vi "Time.vi"(8 "error in (no error)":errorcluster, 10 "Control In":T1={"I-O.lvclass"=refnum, "Motion.lvclass"=refnum, "Dispenser.lvclass"=refnum}, 11 "C4 Dispense in":refnum<class "Iterative Dispense.lvclass">) -> (0 "error out":errorcluster, 1 "Timing Data":i32[](array[numeric]), 2 "Control Out":T1, 3 "C4 Dispense out":refnum<class "Iterative Dispense.lvclass">)   [LabVIEW 2016, in "Iterative Dispense.lvclass"]
uses:
  Iterative Dispense.lvclass
  Controller/Controllers.ctl
  Controller/I-O/I-O.lvclass
  Controller/Motion/A3200/A3200.lvclass
  Controller/Dispenser/Dispenser.lvclass
  Controller/Motion/Motion.lvclass
  Iterative Dispense.lvclass/Iterative Dispense.ctl
  Controller/Controller.lvclass
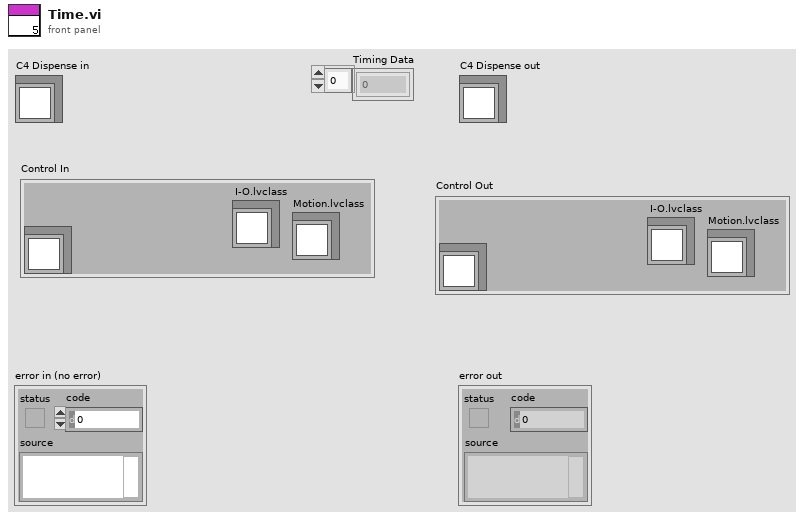
[diagram p1: front panel]
types:
  T1 = typedef "Controller.lvclass/Controllers.ctl" = cluster{"I-O.lvclass":refnum<class "I-O.lvclass">, "Motion.lvclass":refnum<class "Motion.lvclass">, "Dispenser.lvclass":refnum<class "Dispenser.lvclass">}
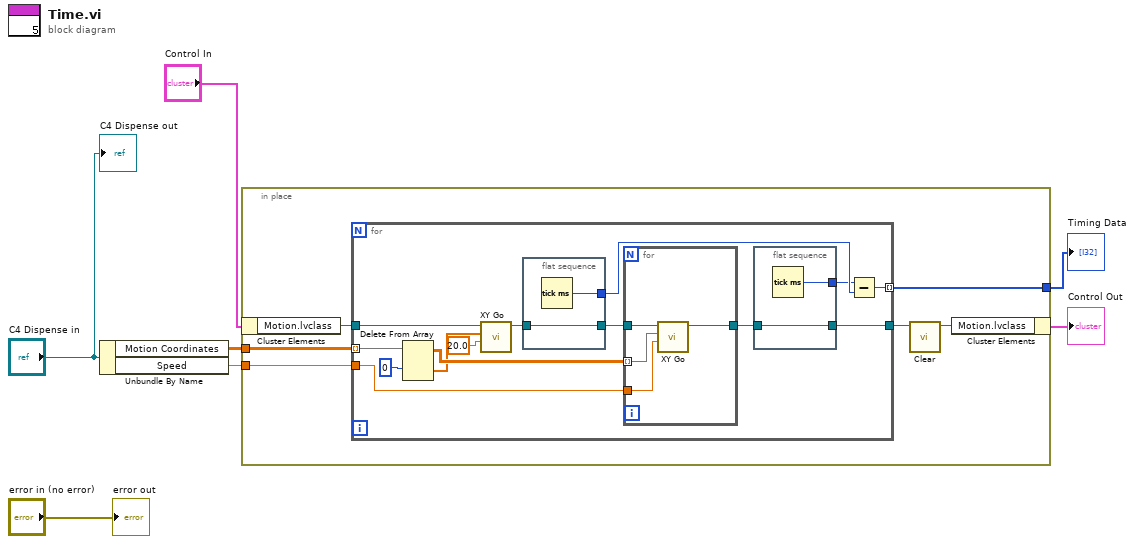
[diagram p0: block diagram]
diagram:
  n1 = Unbundle By Name("C4 Dispense in") -> ("Motion Coordinates"=w7:dbl[][][], "Speed"=w1:dbl)
  n2 = in-place {
    in-place-border: w7 -> [w13]
    in-place-border: [w12] -> w6
    in-place-border: w1 -> [w11]
    n3 = in-place-cluster #1("Control In") -> ("Motion.lvclass"=w10:refnum<class "Motion.lvclass">)
    n4 = for {
      tunnel: [w25] -> w9
      tunnel: [w23] -> w12 mode=indexing
      tunnel: w13 -> [w20] mode=indexing
      tunnel: w11 -> [w19]
      tunnel: w10 -> [w17]
      n5 = Delete From Array(array=w20, index (row)=0) -> (deleted portion=w15:dbl[], array with subset deleted=w22:dbl[][])  [unwired: 2 in]
      n6 = call-dynamic "XY Go.vi"("Speed"=20.0, "XY"=w15, "Motion in"=w17) -> ("Motion out"=w14:refnum<class "Motion.lvclass">)  [unwired: 7 in, 1 out]
      n7 = flat-sequence {
        tunnel: [w31] -> w27
        tunnel: [w30] -> w18
        tunnel: w14 -> [w30]
        frame #0 {
          n8 = Tick Count (ms)() -> (millisecond timer value=w31:u32)
        }
      }
      n9 = for {
        tunnel: [w32] -> w26
        tunnel: w22 -> [w35] mode=indexing
        tunnel: w19 -> [w34]
        tunnel: w18 -> [w33]
        n10 = call-dynamic "XY Go.vi"("Speed"=w34, "XY"=w35, "Motion in"=w33) -> ("Motion out"=w32:refnum<class "Motion.lvclass">)  [unwired: 7 in, 1 out]
      }
      n11 = flat-sequence {
        tunnel: w26 -> [w29]
        tunnel: [w29] -> w25
        tunnel: [w28] -> w24
        frame #0 {
          n12 = Tick Count (ms)() -> (millisecond timer value=w28:u32)
        }
      }
      n13 = Subtract(x=w24, y=w27) -> (x-y=w23:u32)
    }
    n14 = call "Clear.vi"("Motion in"=w9) -> ("Motion out"=w8:refnum<class "Motion.lvclass">)  [unwired: 9 in, 1 out]
    n15 = in-place-cluster #1("Motion.lvclass"=w8) -> (→"Control Out":T1)
  }
  "Timing Data" <- w6
  "error out" <- "error in (no error)"
  "C4 Dispense out" <- "C4 Dispense in"
